vi "button state at index.vi"(9 "not present item indexes":i32[](array[numeric]), 10 "index":i32, 11 "reserved item indexes":i32[](array[numeric])) -> (2 "remove enable":bool, 3 "add enable":bool)   [LabVIEW 2016, in "FPGA Addon System Explorer.lvlib"]
uses:
  FPGA Addon System Explorer.lvlib
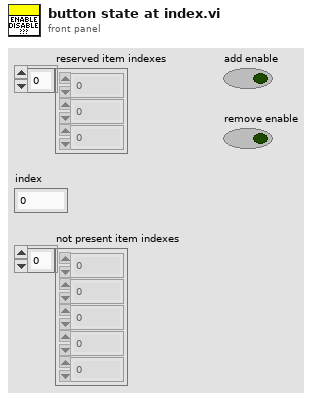
[diagram p1: front panel]
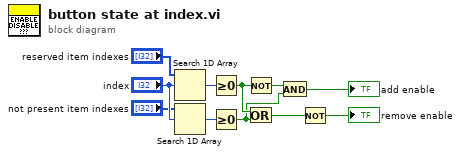
[diagram p0: block diagram]
diagram:
  n1 = Search 1D Array(1D array="reserved item indexes", element="index") -> (index of element=w7:i32)  [unwired: 1 in]
  n2 = Search 1D Array(1D array="not present item indexes", element="index") -> (index of element=w9:i32)  [unwired: 1 in]
  n3 = Greater Or Equal To 0?(x=w7) -> (x >= 0?=w5:bool)
  n4 = Greater Or Equal To 0?(x=w9) -> (x >= 0?=w3:bool)
  n5 = Not(x=w5) -> (.not. x?=w4:bool)
  n6 = Or(x=w5, y=w3) -> (x .or. y?=w6:bool)
  n7 = And(x=w4, y=w3) -> (x .and. y?=→"add enable":bool)
  n8 = Not(x=w6) -> (.not. x?=→"remove enable":bool)
